vi "Update Subsystem.vi"(8 "error in (no error)":errorcluster, 9 "New Owner":refnum<class "Attribute.Owner.lvclass">, 10 "Current Identity":refnum<class "Attribute.Identity.lvclass">) -> (0 "error out":errorcluster, 2 "Updated Identity":refnum<class "Attribute.Identity.lvclass">)   [LabVIEW 2013, in "Registry-SMO.lvclass"]
uses:
  Registry-SMO.lvclass
  Support/Attribute.Owner/Attribute.Owner.lvclass
  Support/Attribute.Identity/Attribute.Identity.lvclass
  SMO_Info--Cluster.ctl
  Support/Attribute.Owner/Attribute.Owner.lvclass/Attribute.Owner.ctl
  Support/Attribute.Identity/Attribute.Identity.lvclass/Attribute.Identity.ctl
  SMO/SMO.lvclass
  Registry-SMO.lvclass/Registry-SMO.ctl
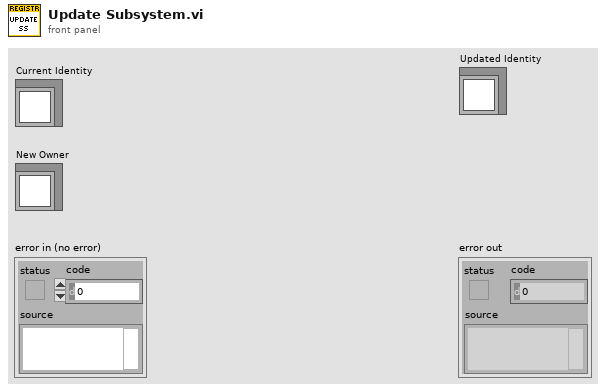
[diagram p1: front panel]
types:
  T1 = typedef "Registry-SMO.lvclass/SMO_Info--Cluster.ctl" = cluster{"Name":string, "Shared Resource":bool}
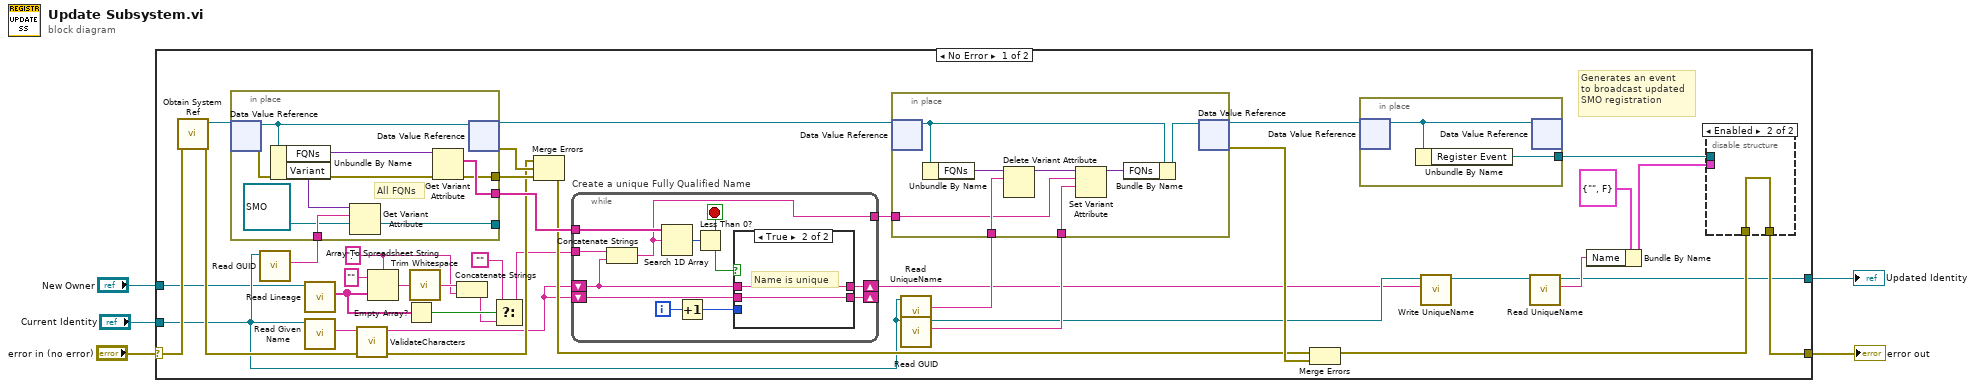
[diagram p0: block diagram]
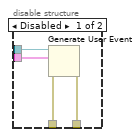
[diagram p2: hidden frame]
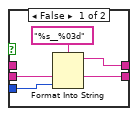
[diagram p3: hidden frame]
diagram:
  n1 = case shown="No Error" "error in (no error)" {
    selector: "error in (no error)" -> [w41 w85]
    tunnel: [w30 w85] -> w4
    tunnel: "New Owner" -> [w19 _]
    tunnel: [w23 w84] -> w2
    tunnel: "Current Identity" -> [w20 w84]
    frame No Error {
      w14 = "." ("delimiter (Tab)")
      # "Generates an event\nto broadcast updated\nSMO registration"
      n2 = call "Obtain System Ref.vi"("error in (no error)"=w41) -> ("error out"=w35:errorcluster, "JKI SMO System"=w40:refnum<data-value>)  [unwired: 9 in]
      n3 = call "Read GUID.vi"("Attribute.Identity in"=w20) -> ("GUID"=w27:string)  [unwired: 8 in, 2 out]
      n4 = in-place {
        in-place-border: [w73] -> w39
        in-place-border: [w72] -> w36
        in-place-border: w27 -> [w69]
        in-place-border: [w67] -> _
        # "All FQNs"
        n5 = in-place-dvr #1(w40) -> (w71:refnum<class "Registry-SMO.lvclass">, w74:errorcluster)
        n6 = Unbundle By Name(w71) -> ("FQNs"=w75:variant, "Variant"=w70:variant)
        n7 = Get Variant Attribute(Variant=w70, name=w69, default value (empty Variant)=refnum<class "SMO.lvclass"> refnum ("SMO")) -> (value=w67:refnum<class "SMO.lvclass">)  [unwired: 1 in, 3 out]
        n8 = Get Variant Attribute(Variant=w75, error in=w74) -> (names=w73:string[], error out=w72:errorcluster)  [unwired: 2 in, 2 out]
        n9 = in-place-dvr #1(w71) -> (w38:refnum<data-value>, w37:errorcluster)
      }
      n10 = call "Read Lineage.vi"("Attribute.Owner in"=w19) -> ("Lineage"=w12:string[])  [unwired: 8 in, 2 out]
      n11 = call "Read Given Name.vi"("Attribute.Identity in"=w20) -> ("Given Name"=w17:string)  [unwired: 9 in, 1 out]
      n12 = call "ValidateCharacters.vi"("Subsystem Name (optional)"=w17) -> ("Validated characters"=w13:string)  [unwired: 10 in]
      n13 = Array To Spreadsheet String(delimiter (Tab)=w14, array=w12, 3:"" ("format string")) -> (spreadsheet string=w16:string)
      n14 = Empty Array?(array=w12) -> (empty?=w11:bool)
      n15 = call <vilib>:"Trim Whitespace.vi"("string"=w16) -> ("trimmed string"=w15:string)  [unwired: 1 in]
      n16 = Concatenate Strings(w15, w14) -> (w10:string)
      n17 = Select(t="", s=w11, f=w10) -> (s? t:f=w9:string)
      n18 = Merge Errors(w35, w37, w36) -> (w34:errorcluster)
      n19 = while "Create a unique Fully Qualified Name" {
        tunnel: w39 -> [w60]
        shift-right: [w57] -> w7
        shift-left: w13 -> [w51]
        shift-right: [w53] -> _
        shift-left: w13 -> [w56]
        tunnel: w9 -> [w52]
        tunnel: [w50] -> w6
        i -> [w55]
        stop <- w58 stop-if-true
        n20 = Concatenate Strings(w52, w51) -> (w50:string)
        n21 = Search 1D Array(1D array=w60, element=w50) -> (index of element=w59:i32)  [unwired: 1 in]
        n22 = Increment(x=w55) -> (x+1=w54:i32)
        n23 = Less Than 0?(x=w59) -> (x < 0?=w58:bool)
        n24 = case shown="True" w58 {
          tunnel: w51 -> [_ w66]
          tunnel: [w64 w66] -> w57
          tunnel: w56 -> [w61 w65]
          tunnel: w54 -> [w63 _]
          tunnel: [w61 w65] -> w53
          frame False {
            n25 = Format Into String(format string="%s__%03d", w61, w63) -> (resulting string=w64:string)  [unwired: 2 in, 1 out]
          }
          frame True {
            # "Name is unique"
          }
        }
      }
      n26 = call "Read UniqueName.vi"("Attribute.Identity in"=w20) -> ("Unique Name"=w26:string)  [unwired: 9 in, 1 out]
      n27 = call "Read GUID.vi"("Attribute.Identity in"=w20) -> ("GUID"=w28:string, "Attribute.Identity out"=w22:refnum<class "Attribute.Identity.lvclass">)  [unwired: 8 in, 1 out]
      n28 = in-place {
        in-place-border: w28 -> [w80]
        in-place-border: w26 -> [w77]
        in-place-border: w6 -> [w76]
        n29 = in-place-dvr #2(w38) -> (w82:refnum<class "Registry-SMO.lvclass">)  [unwired: 1 out]
        n30 = Unbundle By Name(w82) -> ("FQNs"=w79:variant)
        n31 = Delete Variant Attribute(6:w77, 7:w79) -> (3:w78:variant)  [unwired: 1 in, 2 out]
        n32 = Set Variant Attribute(Variant=w78, name=w76, value=w80) -> (Variant out=w81:variant)  [unwired: 1 in, 2 out]
        n33 = Bundle By Name(cluster=w82, "FQNs"=w81) -> (w83:refnum<class "Registry-SMO.lvclass">)
        n34 = in-place-dvr #2(w83) -> (w25:refnum<data-value>, w42:errorcluster)
      }
      n35 = Merge Errors(w34, w42) -> (w24:errorcluster)
      n36 = in-place {
        in-place-border: [w48] -> w33
        n37 = in-place-dvr #3(w25) -> (w49:refnum<class "Registry-SMO.lvclass">)  [unwired: 1 out]
        n38 = Unbundle By Name(w49) -> ("Register Event"=w48:refnum<user-event>)
        n39 = in-place-dvr #3(w49) -> ()  [unwired: 2 out]
      }
      n40 = call "Write UniqueName.vi"("Unique Name"=w7, "Attribute.Identity in"=w22) -> ("Attribute.Identity out"=w21:refnum<class "Attribute.Identity.lvclass">)  [unwired: 9 in]
      n41 = call "Read UniqueName.vi"("Attribute.Identity in"=w21) -> ("Unique Name"=w29:string, "Attribute.Identity out"=w23:refnum<class "Attribute.Identity.lvclass">)  [unwired: 9 in]
      n42 = Bundle By Name(cluster=T1 {"Name"="", "Shared Resource"=FALSE} ("Cluster"), "Name"=w29) -> (w31:T1)
      n43 = disable-structure shown="Enabled" {
        disable-tunnel: w33 -> [w46 _]
        disable-tunnel: w31 -> [w45 _]
        disable-tunnel: [w44 w47] -> w30
        disable-tunnel: w24 -> [w43 w47]
        frame Disabled {
          n44 = Generate User Event(user event=w46, event data cluster=w45, error in=w43) -> (error out=w44:errorcluster)  [unwired: 1 in, 1 out]
        }
        frame Enabled {
        }
      }
    }
    frame Error {
    }
  }
  "error out" <- w4
  "Updated Identity" <- w2
